vi "Encode Base64_2.vi"(1 "string in (not encoded)":string) -> (0 "string out (base64-encoded)":string)   [LabVIEW 2025, in "Encode Base64.lvlib"]
uses:
  Encode Base64.lvlib
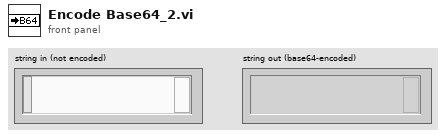
[diagram p1: front panel]
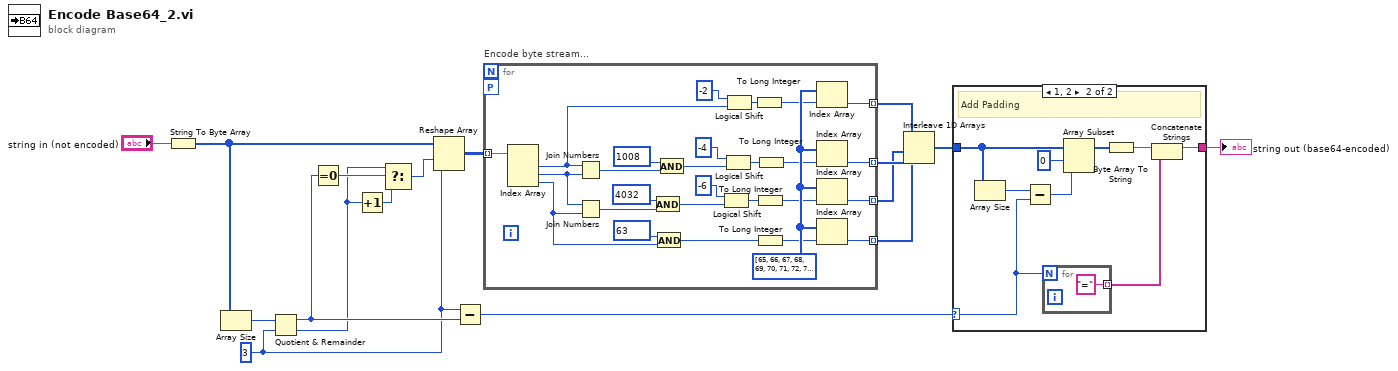
[diagram p0: block diagram]
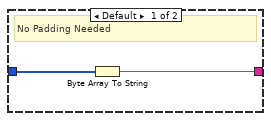
[diagram p2: hidden frame]
diagram:
  w1 = 3 ("y")
  n1 = String To Byte Array(string="string in (not encoded)") -> (unsigned byte array=w5:u8[])
  n2 = Array Size(array=w5) -> (size(s)=w13:i32)
  n3 = Quotient & Remainder(x=w13, y=w1) -> (x-y*floor(x/y)=w14:i32, floor(x/y)=w7:i32)
  n4 = Equal To 0?(x=w14) -> (x = 0?=w15:bool)
  n5 = Increment(x=w7) -> (x+1=w8:i32)
  n6 = Select(t=w7, s=w15, f=w8) -> (s? t:f=w4:i32)
  n7 = Reshape Array(w5, w4, w1) -> (w3:u8[][])
  n8 = Subtract(x=w1, y=w14) -> (x-y=w2:i32)
  n9 = for "Encode byte stream..." {
    tunnel: [w27] -> w9 mode=indexing
    tunnel: [w28] -> w10 mode=indexing
    tunnel: [w29] -> w11 mode=indexing
    tunnel: [w30] -> w12 mode=indexing
    workers-P: _ -> [_]
    tunnel: w3 -> [w21] mode=indexing
    w26 = u8[] [65, 66, 67, 68, 69, 70, 71, 72, 73, 74, 75, 76, 77, 78, 79, 80, 81, 82, 83, 84, 85, 86, 87, 88, 89, 90, 97, 98, 99, 100, 101, 102, 103, 104, 105, 106, 107, 108, 109, 110, 111, 112, 113, 114, 115, 116, 117, 118, 119, 120, 121, 122, 48, 49, 50, 51, 52, 53, 54, 55, 56, 57, 43, 47] ("unsigned byte array")
    n10 = Index Array(array=w21) -> (element #1=w20:u8, element #2=w19:u8, element #3=w18:u8)  [unwired: 3 in]
    n11 = Join Numbers(hi=w20, lo=w19) -> ((hi.lo)=w43:u16)
    n12 = Join Numbers(hi=w19, lo=w18) -> ((hi.lo)=w39:u16)
    n13 = And(x=u16 4032, y=w39) -> (x .and. y?=w37:u16)
    n14 = And(x=u8 63, y=w18) -> (x .and. y?=w31:u8)
    n15 = And(x=u16 1008, y=w43) -> (x .and. y?=w41:u16)
    n16 = Logical Shift(y=i8 -6, x=w37) -> (x << y=w32:u16)
    n17 = Logical Shift(y=i8 -4, x=w41) -> (x << y=w33:u16)
    n18 = Logical Shift(y=i8 -2, x=w20) -> (x << y=w34:u8)
    n19 = To Long Integer(number=w34) -> (32bit integer=w22:i32)
    n20 = To Long Integer(number=w32) -> (32bit integer=w24:i32)
    n21 = To Long Integer(number=w31) -> (32bit integer=w25:i32)
    n22 = To Long Integer(number=w33) -> (32bit integer=w23:i32)
    n23 = Index Array(array=w26, index=w22) -> (element=w30:u8)
    n24 = Index Array(array=w26, index=w23) -> (element=w29:u8)
    n25 = Index Array(array=w26, index=w24) -> (element=w28:u8)
    n26 = Index Array(array=w26, index=w25) -> (element=w27:u8)
  }
  n27 = Interleave 1D Arrays(w12, w11, w10, w9) -> (w6:u8[])
  n28 = case shown="1, 2" w2 {
    selector: w2 -> [_ w51]
    tunnel: [w45 w48] -> w16
    tunnel: w6 -> [w46 w52]
    frame Default {
      # "No Padding Needed"
      n29 = Byte Array To String(unsigned byte array=w46) -> (string=w45:string)
    }
    frame 1, 2 {
      # "Add Padding"
      n30 = Array Size(array=w52) -> (size(s)=w53:i32)
      n31 = Subtract(x=w53, y=w51) -> (x-y=w49:i32)
      n32 = for {
        N: w51 -> [_]
        tunnel: ["="] -> w47 mode=indexing
      }
      n33 = Array Subset(array=w52, index=0, length=w49) -> (w55:u8[])
      n34 = Byte Array To String(unsigned byte array=w55) -> (string=w54:string)
      n35 = Concatenate Strings(w54, w47) -> (w48:string)
    }
  }
  "string out (base64-encoded)" <- w16
